vi "String To Path.vi"(6 "Default":path, 8 "error in (no error)":errorcluster, 10 "String":string, 11 "Registry Object":refnum<class "Carya Config.lvclass">) -> (0 "error out":errorcluster, 2 "Path":path, 3 "Registry Object":refnum<class "Carya Config.lvclass">)   [LabVIEW 2013, in "Carya Config.lvclass"]
doc: "Copyright 2018, Carya Automatisering, Wiebe Walstra."
uses:
  Carya Config.lvclass
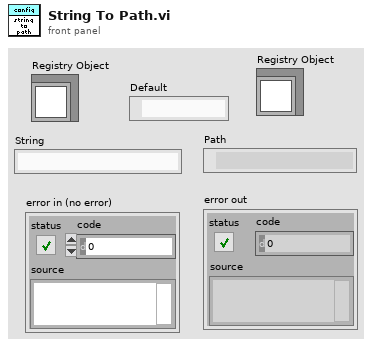
[diagram p1: front panel]
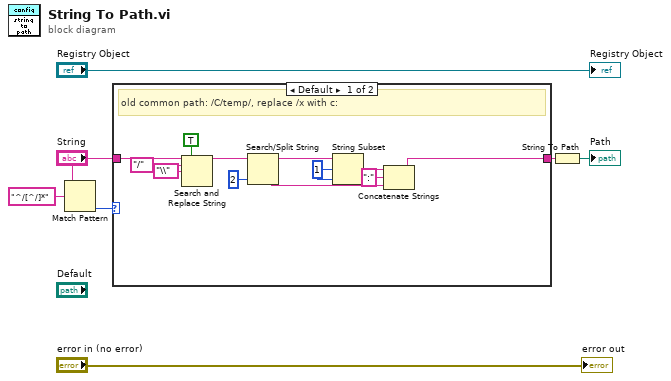
[diagram p0: block diagram]
diagram:
  n1 = Match Pattern(string="String", regular expression="^/[^/]*") -> (offset past match=w1:i32)  [unwired: 1 in, 3 out]
  n2 = case shown="Default" w1 {
    tunnel: [w19 w20] -> w5
    tunnel: "String" -> [w14 w20]
    frame Default {
      w8 = 1 ("offset (0)")
      # "old common path: /C/temp/, replace /x with c:"
      n3 = Search and Replace String(replace all?=TRUE ("replace all? (F)"), input string=w14, search string="/", replace string="\\" ("replace string (\"\")")) -> (result string=w15:string)  [unwired: 4 in, 3 out]
      n4 = Search/Split String(string=w15, offset (0)=2) -> (substring before match=w12:string, match + rest of string=w9:string)  [unwired: 2 out]
      n5 = String Subset(string=w12, offset (0)=w8, length (rest)=w8) -> (substring=w11:string)
      n6 = Concatenate Strings(w11, ":", w9) -> (w19:string)
    }
    frame -1 {
    }
  }
  n7 = String To Path(string=w5) -> (path=→"Path":path)
  "Registry Object" <- "Registry Object"
  "error out" <- "error in (no error)"
